vi "VS-Read Heart Rate.vi"(8 "error in (no error)":errorcluster) -> (0 "error out":errorcluster, 2 "Temp (C)":dbl format="%.1f")   [LabVIEW 2020]
uses:
  Connection Manager/Type Defs/Input sources.ctl
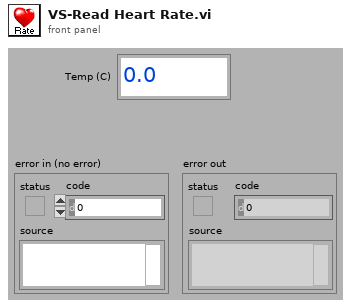
[diagram p1: front panel]
types:
  T1 = typedef "Input sources.ctl" = u16
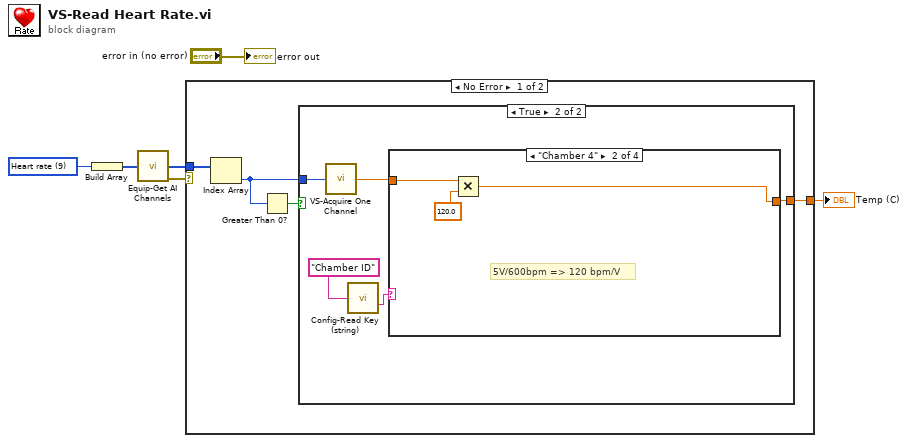
[diagram p0: block diagram]
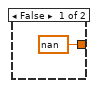
[diagram p2: hidden frame]
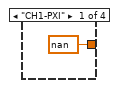
[diagram p3: hidden frame]
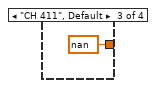
[diagram p4: hidden frame]
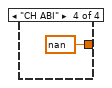
[diagram p5: hidden frame]
diagram:
  w5 = T1 9 items=["--unused--", "Probe Mic Right", "Probe Mic Left", "Cal Mic", "ABR", "CAP Right", "CAP Left", "Startle piezo", "Temperature", "Heart rate"] ("Ring")
  n1 = Build Array(w5) -> (w4:T1[])
  n2 = call "Equip-Get AI Channels.vi"("Inputs"=w4) -> ("AI Channels"=w3:i32[], "error out"=w2:errorcluster)  [unwired: 13 in]
  n3 = case shown="No Error" w2 {
    tunnel: [w10 _] -> w6
    tunnel: w3 -> [w9 _]
    frame No Error {
      n4 = Index Array(array=w9) -> (element=w8:i32)  [unwired: 1 in]
      n5 = Greater Than 0?(x=w8) -> (x > 0?=w7:bool)
      n6 = case shown="True" w7 {
        tunnel: [nan w16] -> w10
        tunnel: w8 -> [_ w14]
        frame False {
        }
        frame True {
          n7 = call "VS-Acquire One Channel.vi"("index"=w14) -> ("mean"=w15:dbl)  [unwired: 13 in, 1 out]
          n8 = call "Config-Read Key (string).vi"("key"="Chamber ID" ("string")) -> ("value"=w12:string)  [unwired: 11 in, 3 out]
          n9 = case shown="\"Chamber 4\"" w12 {
            tunnel: w15 -> [_ w19 _ _]
            tunnel: [nan w18 nan nan] -> w16
            frame "CH1-PXI" {
            }
            frame "Chamber 4" {
              # "5V/600bpm => 120 bpm/V"
              n10 = Multiply(x=w19, y=120.0) -> (x*y=w18:dbl)
            }
            frame "CH 411", Default {
            }
            frame "CH ABI" {
            }
          }
        }
      }
    }
    frame Error {
    }
  }
  "Temp (C)" <- w6
  "error out" <- "error in (no error)"
